vi "Problem 2 - Even Fibonacci numbers.vi"() -> ()   [LabVIEW 2021, in "Project Euler.lvlib"]
uses:
  Project Euler.lvlib
  Utilities/Numeric Utilities/Numeric Utilities.lvlib
panel:
  out "Answer":i32
  out "Even Fibonacci terms <= 4,000,000":i32[](array[numeric])
  # "Development\nControls or indicators that are useful for development or testing, but which are not outputs of the VI."
  # "Input\nInputs to the VI"
  # "Output\nOutputs of the VI"
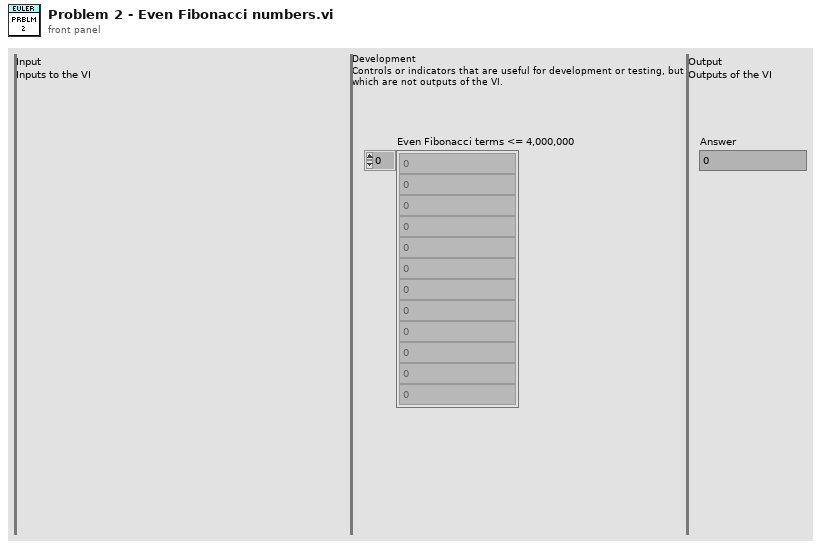
[diagram p1: front panel]
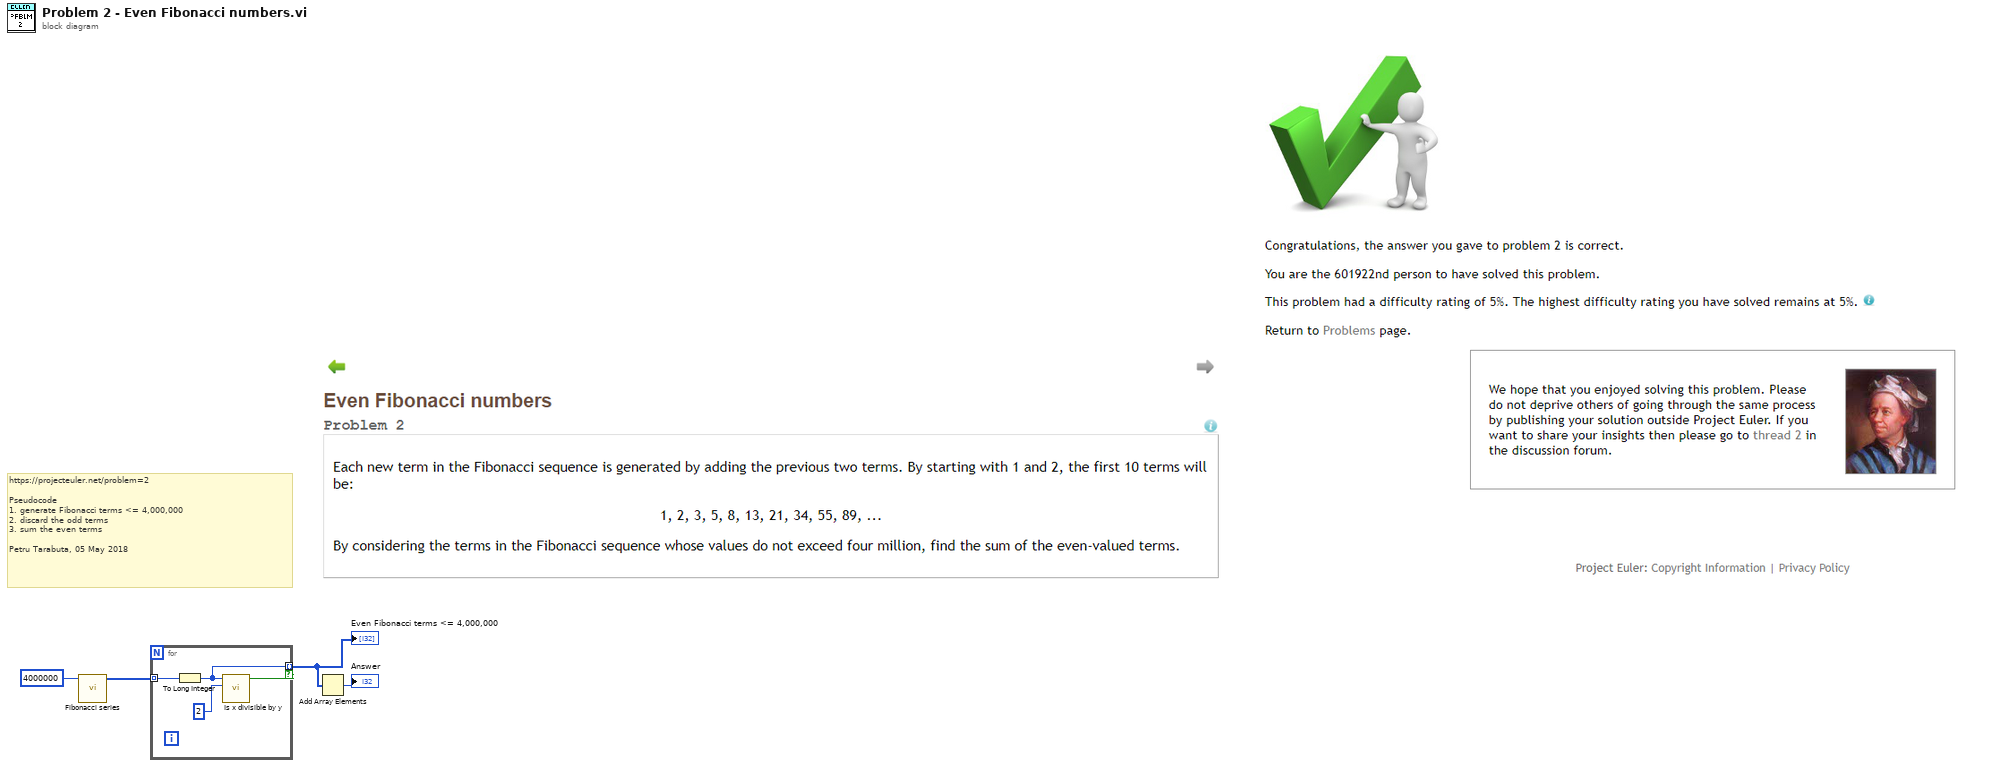
[diagram p0: block diagram]
diagram:
  # "https://projecteuler.net/problem=2\n\nPseudocode\n1. generate Fibonacci terms <= 4,000,000\n2. discard the odd terms\n3. sum the even terms\n\nPetru Tarabuta, 05 May 2018"
  n1 = call "Fibonacci series.vi"("Generate Fibonacci terms that are <= this number (dflt=one million)"=u64 4000000) -> ("Fibonacci series"=w3:u64[])  [unwired: 8 in, 2 out]
  n2 = for {
    tunnel: w3 -> [w8] mode=indexing
    tunnel: [w6] -> w2 mode=indexing if=w5
    n3 = To Long Integer(number=w8) -> (32bit integer=w6:i32)
    n4 = call "Is x divisible by y.vi"("y"=2, "x"=w6) -> ("T = x is divisible by y"=w5:bool)  [unwired: 7 in, 2 out]
  }
  "Even Fibonacci terms <= 4,000,000" <- w2
  n5 = Add Array Elements(numeric array=w2) -> (sum=→"Answer":i32)
